vi "AMI430_Magnet controller Interface_PK.vi"() -> ()   [LabVIEW 2016]
panel:
  in  "Y-AXIS ON/OFF":bool=TRUE
  in  "Z-AXIS ON/OFF":bool=TRUE
  in  "Y-Axis Magnet IP Address":string="169.254.67.34"
  out "Y-axis Magnetic Field (T)":string="0.000010141\r\n"
  out "Y-axis Target Field (T)":string="0.000000000\r\n"
  out "Y-axis Ramp rate (T/min)":dbl=0.005 format="%#_13g"
  in  "Y-AXIS\nRAMP":bool
  in  "Y-axis Target Field setpoint (T)":string="0"
  in  "Y-axis Ramp Rate (T/min)":string="0.005"
  out "Z-axis Magnetic Field (T)":string="-0.000034406\r\n"
  out "Z-axis Target Field (T)":string="0.000000000\r\n"
  out "Z-axis Ramp rate (T/min)":dbl=0.005 format="%#_13g"
  in  "Z-axis Target Field setpoint (T)":string="0"
  in  "Z-axis Ramp Rate (T/min)":string="0.005"
  in  "Z-AXIS\nRAMP":bool
  in  "Z-Axis Magnet IP Address":string="169.254.207.70"
  in  "?":bool
  # "AMI 430 Magnet controller Interface\nfor Bluefors LD-400 - PK v1.0\nZ-Axis: In-plane\nY-axis: Out-of-plane"
  # "PAUSE"
  # "PAUSE"
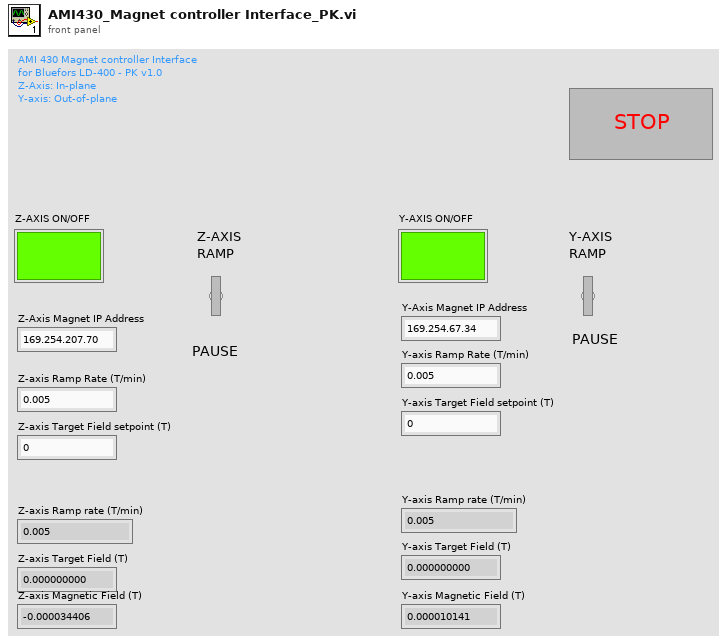
[diagram p1: front panel]
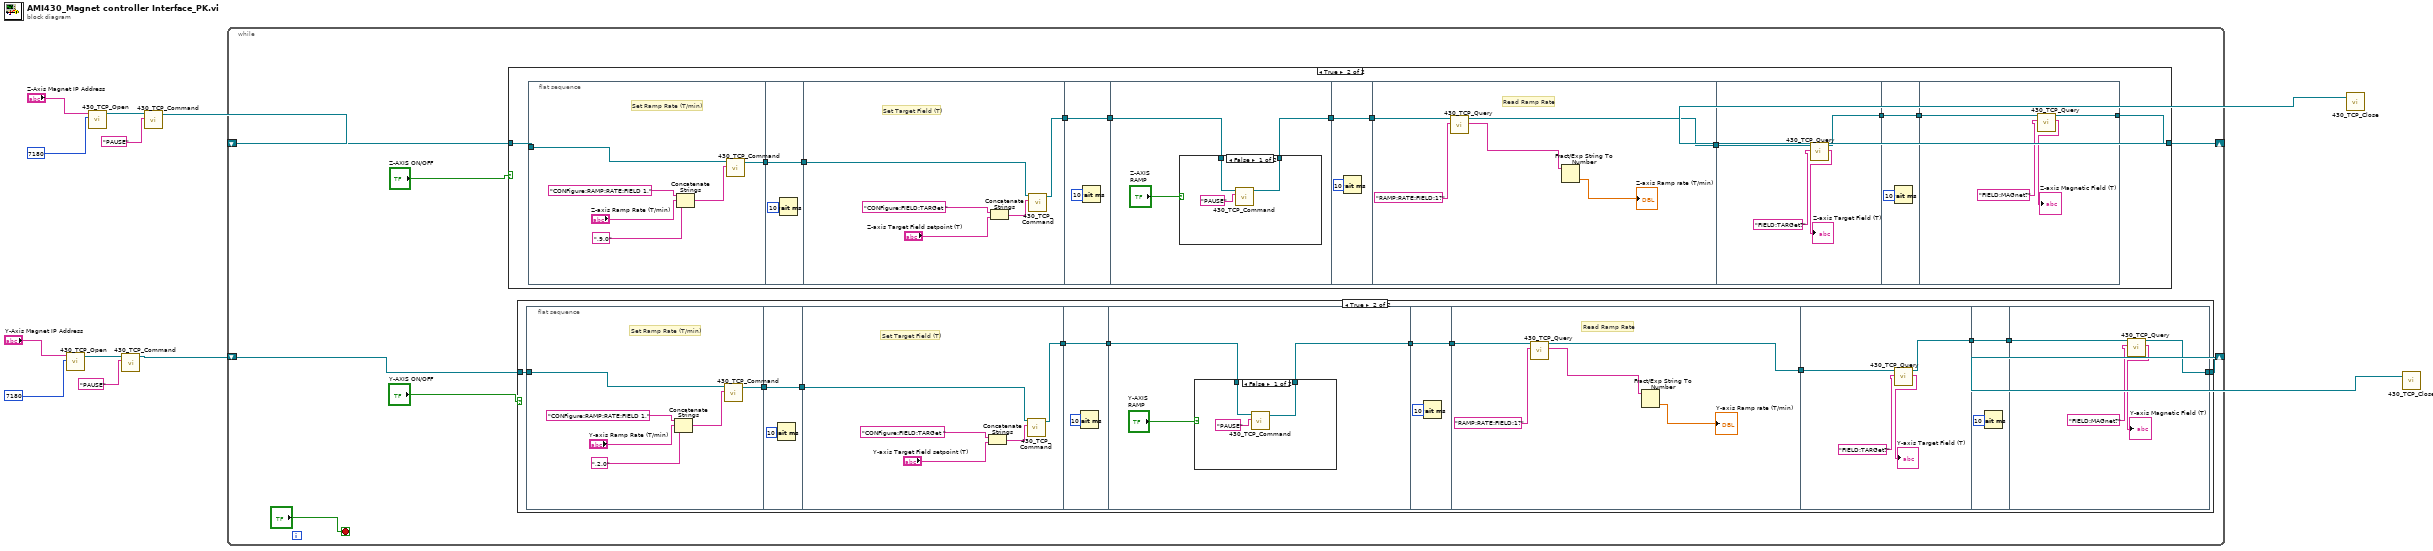
[diagram p0: block diagram]
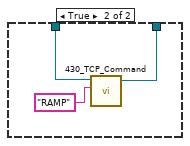
[diagram p3: hidden frame]
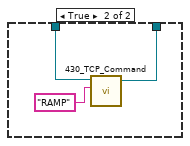
[diagram p5: hidden frame]
diagram:
  n1 = call "430_TCP_Open.vi"("IP Address"="Y-Axis Magnet IP Address", "TCP Port"=7180) -> ("connection ID"=w5:refnum<k5>)  [unwired: 4 in, 2 out]
  n2 = call "430_TCP_Open.vi"("IP Address"="Z-Axis Magnet IP Address", "TCP Port"=7180) -> ("connection ID"=w10:refnum<k5>)  [unwired: 4 in, 2 out]
  n3 = call "430_TCP_Command.vi"("Command"="PAUSE", "connection ID"=w5) -> ("connection ID out"=w3:refnum<k5>)  [unwired: 2 in, 2 out]
  n4 = call "430_TCP_Command.vi"("Command"="PAUSE", "connection ID"=w10) -> ("connection ID out"=w8:refnum<k5>)  [unwired: 2 in, 2 out]
  n5 = while {
    shift-right: [w13] -> w2
    shift-left: w8 -> [w18]
    shift-right: [w16] -> w1
    shift-left: w3 -> [w17]
    stop <- "?" stop-if-true
    n6 = case shown="True" "Z-AXIS ON/OFF" {
      tunnel: w18 -> [w20 w22]
      tunnel: [w20 w21] -> w13
      frame False {
      }
      frame True {
        n7 = flat-sequence {
          tunnel: w22 -> [w37]
          tunnel: [w32] -> w31
          tunnel: w31 -> [w39]
          tunnel: [w39] -> w30
          tunnel: w30 -> [w41]
          tunnel: [w40] -> w29
          tunnel: [w45] -> w28
          tunnel: w29 -> [w45]
          tunnel: [w47] -> w27
          tunnel: w28 -> [w48]
          tunnel: w27 -> [w57]
          tunnel: [w57] -> w26
          tunnel: w26 -> [w61]
          tunnel: [w58] -> w25
          tunnel: w25 -> [w65]
          tunnel: [w63] -> w24
          tunnel: [w68] -> w23
          tunnel: w24 -> [w68]
          tunnel: w23 -> [w70]
          tunnel: [w69] -> w21
          frame #0 {
            # "Set Ramp Rate (T/min)"
            n8 = Concatenate Strings("CONFigure:RAMP:RATE:FIELD 1,", "Z-axis Ramp Rate (T/min)", ",9.0") -> (w33:string)
            n9 = call "430_TCP_Command.vi"("Command"=w33, "connection ID"=w37) -> ("connection ID out"=w32:refnum<k5>)  [unwired: 2 in, 2 out]
          }
          frame #1 {
            n10 = Wait (ms)(milliseconds to wait=10) -> ()  [unwired: 1 out]
          }
          frame #2 {
            # "Set Target Field (T)"
            n11 = Concatenate Strings("CONFigure:FIELD:TARGet ", "Z-axis Target Field setpoint (T)") -> (w42:string)
            n12 = call "430_TCP_Command.vi"("Command"=w42, "connection ID"=w41) -> ("connection ID out"=w40:refnum<k5>)  [unwired: 2 in, 2 out]
          }
          frame #3 {
            n13 = Wait (ms)(milliseconds to wait=10) -> ()  [unwired: 1 out]
          }
          frame #4 {
            n14 = case shown="False" "Z-AXIS\nRAMP" {
              tunnel: w48 -> [w52 w55]
              tunnel: [w50 w53] -> w47
              frame False {
                n15 = call "430_TCP_Command.vi"("Command"="PAUSE", "connection ID"=w52) -> ("connection ID out"=w50:refnum<k5>)  [unwired: 2 in, 2 out]
              }
              frame True {
                n16 = call "430_TCP_Command.vi"("Command"="RAMP", "connection ID"=w55) -> ("connection ID out"=w53:refnum<k5>)  [unwired: 2 in, 2 out]
              }
            }
          }
          frame #5 {
            n17 = Wait (ms)(milliseconds to wait=10) -> ()  [unwired: 1 out]
          }
          frame #6 {
            # "Read Ramp Rate"
            n18 = call "430_TCP_Query.vi"("Command"="RAMP:RATE:FIELD:1?" ("Magnetic Field (T)"), "connection ID"=w61) -> ("Response"=w59:string, "connection ID out"=w58:refnum<k5>)  [unwired: 5 in, 3 out]
            n19 = Fract/Exp String To Number(string=w59) -> (number=→"Z-axis Ramp rate (T/min)":dbl)  [unwired: 3 in, 1 out]
          }
          frame #7 {
            n20 = call "430_TCP_Query.vi"("Command"="FIELD:TARGet?" ("Magnetic Field (T)"), "connection ID"=w65) -> ("Response"=→"Z-axis Target Field (T)":string, "connection ID out"=w63:refnum<k5>)  [unwired: 5 in, 3 out]
          }
          frame #8 {
            n21 = Wait (ms)(milliseconds to wait=10) -> ()  [unwired: 1 out]
          }
          frame #9 {
            n22 = call "430_TCP_Query.vi"("Command"="FIELD:MAGnet?" ("Magnetic Field (T)"), "connection ID"=w70) -> ("Response"=→"Z-axis Magnetic Field (T)":string, "connection ID out"=w69:refnum<k5>)  [unwired: 5 in, 3 out]
          }
        }
      }
    }
    n23 = case shown="True" "Y-AXIS ON/OFF" {
      tunnel: w17 -> [w73 w75]
      tunnel: [w73 w74] -> w16
      frame False {
      }
      frame True {
        n24 = flat-sequence {
          tunnel: w75 -> [w90]
          tunnel: [w85] -> w84
          tunnel: w84 -> [w92]
          tunnel: [w92] -> w83
          tunnel: w83 -> [w94]
          tunnel: [w93] -> w82
          tunnel: [w98] -> w81
          tunnel: w82 -> [w98]
          tunnel: [w100] -> w80
          tunnel: w81 -> [w101]
          tunnel: w80 -> [w110]
          tunnel: [w110] -> w79
          tunnel: w79 -> [w114]
          tunnel: [w111] -> w78
          tunnel: w78 -> [w118]
          tunnel: [w116] -> w77
          tunnel: [w121] -> w76
          tunnel: w77 -> [w121]
          tunnel: w76 -> [w123]
          tunnel: [w122] -> w74
          frame #0 {
            # "Set Ramp Rate (T/min)"
            n25 = Concatenate Strings("CONFigure:RAMP:RATE:FIELD 1,", "Y-axis Ramp Rate (T/min)", ",2.0") -> (w86:string)
            n26 = call "430_TCP_Command.vi"("Command"=w86, "connection ID"=w90) -> ("connection ID out"=w85:refnum<k5>)  [unwired: 2 in, 2 out]
          }
          frame #1 {
            n27 = Wait (ms)(milliseconds to wait=10) -> ()  [unwired: 1 out]
          }
          frame #2 {
            # "Set Target Field (T)"
            n28 = Concatenate Strings("CONFigure:FIELD:TARGet ", "Y-axis Target Field setpoint (T)") -> (w95:string)
            n29 = call "430_TCP_Command.vi"("Command"=w95, "connection ID"=w94) -> ("connection ID out"=w93:refnum<k5>)  [unwired: 2 in, 2 out]
          }
          frame #3 {
            n30 = Wait (ms)(milliseconds to wait=10) -> ()  [unwired: 1 out]
          }
          frame #4 {
            n31 = case shown="False" "Y-AXIS\nRAMP" {
              tunnel: w101 -> [w105 w108]
              tunnel: [w103 w106] -> w100
              frame False {
                n32 = call "430_TCP_Command.vi"("Command"="PAUSE", "connection ID"=w105) -> ("connection ID out"=w103:refnum<k5>)  [unwired: 2 in, 2 out]
              }
              frame True {
                n33 = call "430_TCP_Command.vi"("Command"="RAMP", "connection ID"=w108) -> ("connection ID out"=w106:refnum<k5>)  [unwired: 2 in, 2 out]
              }
            }
          }
          frame #5 {
            n34 = Wait (ms)(milliseconds to wait=10) -> ()  [unwired: 1 out]
          }
          frame #6 {
            # "Read Ramp Rate"
            n35 = call "430_TCP_Query.vi"("Command"="RAMP:RATE:FIELD:1?" ("Magnetic Field (T)"), "connection ID"=w114) -> ("Response"=w112:string, "connection ID out"=w111:refnum<k5>)  [unwired: 5 in, 3 out]
            n36 = Fract/Exp String To Number(string=w112) -> (number=→"Y-axis Ramp rate (T/min)":dbl)  [unwired: 3 in, 1 out]
          }
          frame #7 {
            n37 = call "430_TCP_Query.vi"("Command"="FIELD:TARGet?" ("Magnetic Field (T)"), "connection ID"=w118) -> ("Response"=→"Y-axis Target Field (T)":string, "connection ID out"=w116:refnum<k5>)  [unwired: 5 in, 3 out]
          }
          frame #8 {
            n38 = Wait (ms)(milliseconds to wait=10) -> ()  [unwired: 1 out]
          }
          frame #9 {
            n39 = call "430_TCP_Query.vi"("Command"="FIELD:MAGnet?" ("Magnetic Field (T)"), "connection ID"=w123) -> ("Response"=→"Y-axis Magnetic Field (T)":string, "connection ID out"=w122:refnum<k5>)  [unwired: 5 in, 3 out]
          }
        }
      }
    }
  }
  n40 = call "430_TCP_Close.vi"("connection ID"=w2) -> ()  [unwired: 1 in, 2 out]
  n41 = call "430_TCP_Close.vi"("connection ID"=w1) -> ()  [unwired: 1 in, 2 out]
